vi "WPI_DigitalModuleDIOAllocator.vi"(7 "AllocatedDIOMutex":T2, 8 "error in (no error)":errorcluster, 9 "Input? (F)":bool, 10 "DIOChannel":T1=enum."DIO 1") -> (0 "error out":errorcluster, 2 "Allocated DIOChannel":T1=enum."DIO 1", 3 "AllocatedDIO":bool)   [LabVIEW 2017]
doc: "This software is licensed. Open the labview\\readme\\WPI Robotics Library Open Source License.txt file for more information."
uses:
  <vilib>/Rock Robotics/SystemInterfaces/DIO/FPGA_DIOChannel.ctl
  <vilib>/Rock Robotics/WPI/DigitalModule/WPI_DigitalModuleDIOCacheOp.ctl
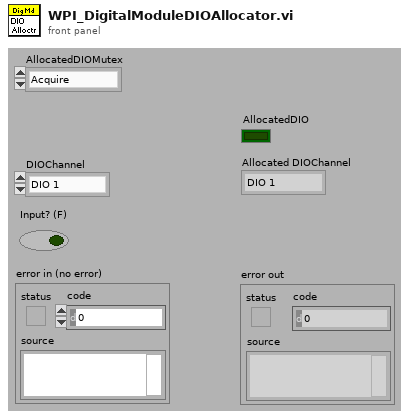
[diagram p1: front panel]
types:
  T1 = typedef "FPGA_DIOChannel.ctl" = enum8{"DIO 0", "DIO 1", "DIO 2", "DIO 3", "DIO 4", "DIO 5", "DIO 6", "DIO 7", "DIO 8", "DIO 9", "DIO MXP 0", "DIO MXP 1", "DIO MXP 2", "DIO MXP 3", "DIO MXP 4", "DIO MXP 5", "DIO MXP 6", "DIO MXP 7", "DIO MXP 8", "DIO MXP 9", "DIO MXP 10", "DIO MXP 11", "DIO MXP 12", "DIO MXP 13", "DIO MXP 14", "DIO MXP 15", "SPI Port CS1", "SPI Port CS2", "SPI Port CS3", "SPI Port MISO", "SPI Port MOSI", "Invalid"}
  T2 = typedef "WPI_DigitalModuleDIOCacheOp.ctl" = enum16{"Acquire", "Release", "Status"}
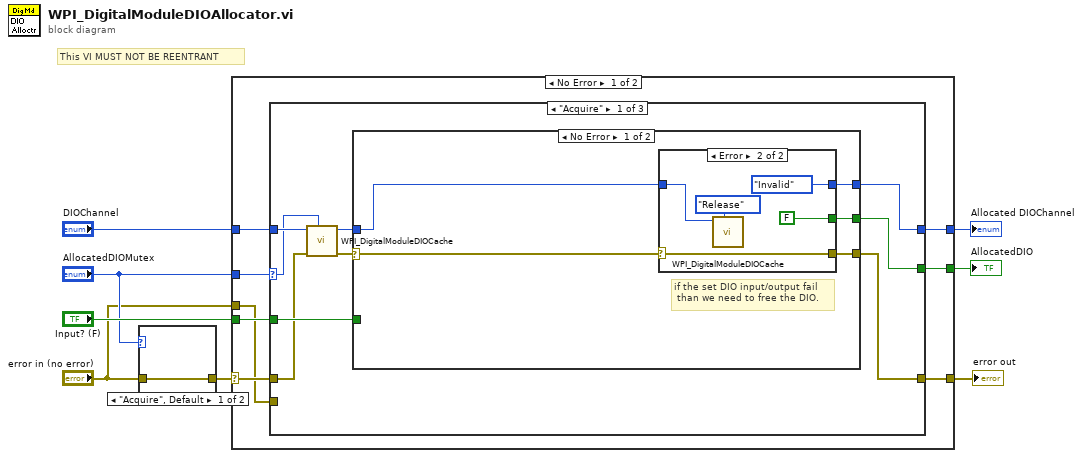
[diagram p0: block diagram]
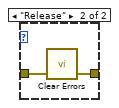
[diagram p2: hidden frame]
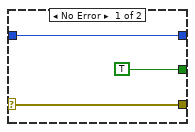
[diagram p3: hidden frame]
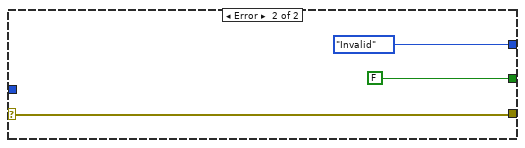
[diagram p4: hidden frame]
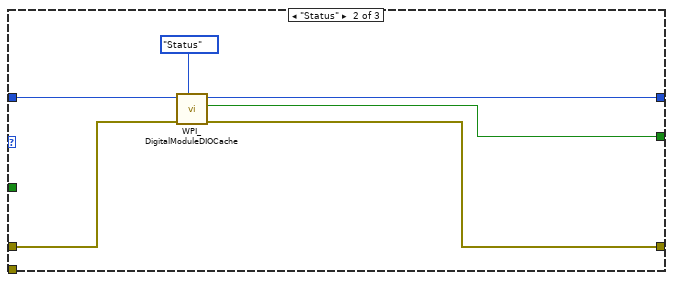
[diagram p5: hidden frame]
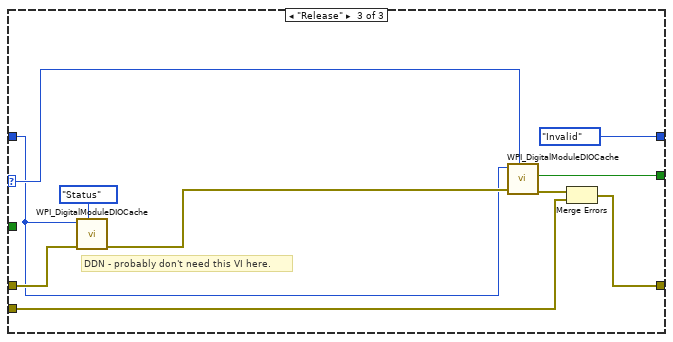
[diagram p6: hidden frame]
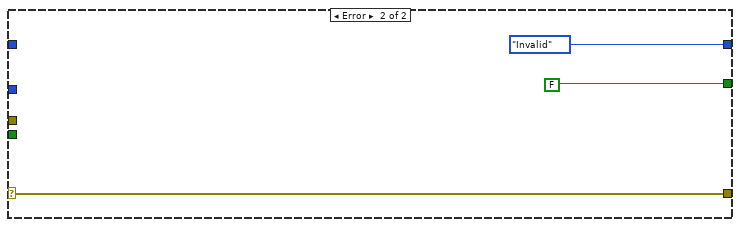
[diagram p7: hidden frame]
diagram:
  # "This VI MUST NOT BE REENTRANT"
  n1 = case shown="\"Acquire\", Default" "AllocatedDIOMutex" {
    tunnel: "error in (no error)" -> [w9 w11]
    tunnel: [w9 w10] -> w6
    frame "Acquire", Default {
    }
    frame "Release" {
      n2 = call <vilib>:"Clear Errors.vi"("error in (no error)"=w11) -> ("error out"=w10:errorcluster)  [unwired: 1 in, 5 out]
    }
  }
  n3 = case shown="No Error" w6 {
    selector: w6 -> [w17 w62]
    tunnel: "Input? (F)" -> [w19 _]
    tunnel: "DIOChannel" -> [w15 _]
    tunnel: [w18 FALSE ("Allocated")] -> w5
    tunnel: [w16 w62] -> w1
    tunnel: "AllocatedDIOMutex" -> [w14 _]
    tunnel: [w13 FPGA_DIOChannel."Invalid" ("DIOChannel Allocated")] -> w4
    tunnel: "error in (no error)" -> [w12 _]
    frame No Error {
      n4 = case shown="\"Acquire\"" w14 {
        selector: w14 -> [w21 _ w57]
        tunnel: w19 -> [w28 _ _]
        tunnel: [w27 w46 w55] -> w18
        tunnel: w17 -> [w25 w48 w60]
        tunnel: [w24 w47 w51] -> w16
        tunnel: w15 -> [w23 w50 w56]
        tunnel: [w20 w45 FPGA_DIOChannel."Invalid" ("DIOChannel Allocated")] -> w13
        tunnel: w12 -> [_ _ w53]
        frame "Acquire" {
          n5 = call <vilib>:"WPI_DigitalModuleDIOCache.vi"("Operation"=w21, "error in (no error)"=w25, "DIOChannel"=w23) -> ("error out"=w26:errorcluster, "DIOChannel Allocated"=w22:T1)  [unwired: 2 in, 5 out]
          n6 = case shown="No Error" w26 {
            selector: w26 -> [w29 w44]
            tunnel: w22 -> [w30 _]
            tunnel: w28 -> [_ _]
            tunnel: [w32 w44] -> w24
            tunnel: [w33 FALSE] -> w27
            tunnel: [w31 FPGA_DIOChannel."Invalid" ("DIOChannel Allocated")] -> w20
            frame No Error {
              # "if the set DIO input/output fail\n than we need to free the DIO."
              n7 = case shown="Error" w29 {
                selector: w29 -> [w35 w37]
                tunnel: [w35 w37] -> w32
                tunnel: w30 -> [w34 w40]
                tunnel: [TRUE FALSE] -> w33
                tunnel: [w34 FPGA_DIOChannel."Invalid" ("DIOChannel Allocated")] -> w31
                frame No Error {
                }
                frame Error {
                  n8 = call <vilib>:"WPI_DigitalModuleDIOCache.vi"("Operation"=WPI_DigitalModuleDIOCacheOp."Release", "DIOChannel"=w40) -> ()  [unwired: 3 in, 7 out]
                }
              }
            }
            frame Error {
            }
          }
        }
        frame "Status" {
          n9 = call <vilib>:"WPI_DigitalModuleDIOCache.vi"("Operation"=WPI_DigitalModuleDIOCacheOp."Status", "error in (no error)"=w48, "DIOChannel"=w50) -> ("error out"=w47:errorcluster, "Allocated"=w46:bool, "DIOChannel Allocated"=w45:T1)  [unwired: 1 in, 5 out]
        }
        frame "Release" {
          # "DDN - probably don't need this VI here."
          n10 = call <vilib>:"WPI_DigitalModuleDIOCache.vi"("Operation"=WPI_DigitalModuleDIOCacheOp."Status", "error in (no error)"=w60, "DIOChannel"=w56) -> ("error out"=w58:errorcluster)  [unwired: 1 in, 7 out]
          n11 = call <vilib>:"WPI_DigitalModuleDIOCache.vi"("Operation"=w57, "error in (no error)"=w58, "DIOChannel"=w56) -> ("error out"=w52:errorcluster, "Allocated"=w55:bool)  [unwired: 1 in, 6 out]
          n12 = Merge Errors(w52, w53) -> (w51:errorcluster)
        }
      }
    }
    frame Error {
    }
  }
  "AllocatedDIO" <- w5
  "error out" <- w1
  "Allocated DIOChannel" <- w4
